vi "PH_ForceSensor.PC Write PSDB.vi"(0 "i ref in":refnum<vi>, 5 "error IO":errorcluster) -> (14 "i ref out":refnum<vi>, 19 "error out":errorcluster)   [LabVIEW 2014, in "PH_ForceSensor.lvlib"]
doc: "This is the proc case which writes data to the PHELIX shot data base."
uses:
  PH_ForceSensor.lvlib
  PH_Basics/PH_PSDBWriter/PH_PSDBWriter.lvlib
  PH_Basics/PH_StatusHandler/PH_StatusHandler.lvlib
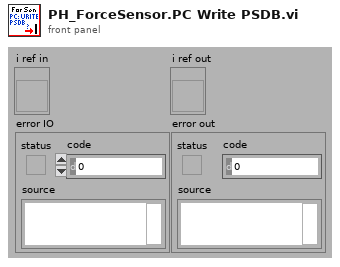
[diagram p1: front panel]
types:
  T1 = typedef "PH_PSDBWriter.lvlib/PH_PSDBWriter.String dataset.ctl" = cluster{"name":string, "data":string, "unit":string}
  T2 = typedef "PH_ForceSensor.lvlib/PH_ForceSensor.i attribute.ctl" = cluster{"GUI Refs":T3, "Rawvalues":T4, "Offsets [µV]":T4, "Scalings [mV/V]":T4, "Forces [N]":T4, "Supply Voltage [V]":dbl, "Full Force [N]":dbl, "Ranges [N]":cluster{"Low Energy":cluster{"Upper Limit":dbl, "Lower Limit":dbl}, "High Energy":cluster{"Upper Limit":dbl, "Lower Limit":dbl}}}
  T3 = typedef "PH_ForceSensor.lvlib/PH_ForceSensor.GUI Refs.ctl" = cluster{"Delete":refnum<vi>, "Rawvalues":refnum<vi>, "Offsets [µV]":refnum<vi>, "Sensor Values [µV]":refnum<vi>, "Scalings [mV/V]":refnum<vi>, "Supply Voltage [V]":refnum<vi>, "Full Force [N]":refnum<vi>, "Forces [N]":refnum<vi>, "Graph Differential Forces":refnum<vi>, "Graph Absolute Forces":refnum<vi>, "Ranges [N]":refnum<vi>}
  T4 = typedef "PH_ForceSensor.lvlib/PH_ForceSensor.Dataset.ctl" = cluster{"top front":dbl, "top back":dbl, "bottom front":dbl, "bottom back":dbl}
  T5 = typedef "PH_PSDBWriter.lvlib/PH_PSDBWriter.Numeric dataset.ctl" = cluster{"name":string, "data":dbl, "unit":string}
  T6 = typedef "PH_PSDBWriter.lvlib/PH_PSDBWriter.PSDB Dataset.ctl" = cluster{"Version":i32, "2D data Input":T7[], "Boolean Input":T9[], "Image Input":T10[], "Numeric Input":T5[], "String Input":T1[]}
  T7 = typedef "PH_PSDBWriter.lvlib/PH_PSDBWriter.2D dataset.ctl" = cluster{"name":string, "data":dbl[][], "axis description":T8}
  T8 = typedef "PSDB.lvlib/PSDB_AxisDescription.ctl" = cluster{"x axis label":string, "y axis label":string, "x axis unit":string, "y axis unit":string}
  T9 = typedef "PH_PSDBWriter.lvlib/PH_PSDBWriter.Boolean dataset.ctl" = cluster{"name":string, "data":bool, "unit":string}
  T10 = typedef "PH_PSDBWriter.lvlib/PH_PSDBWriter.Image dataset.ctl" = cluster{"name":string, "data":T11, "unit":string}
  T11 = typedef "IMAQ Image.ctl" = refnum<image>
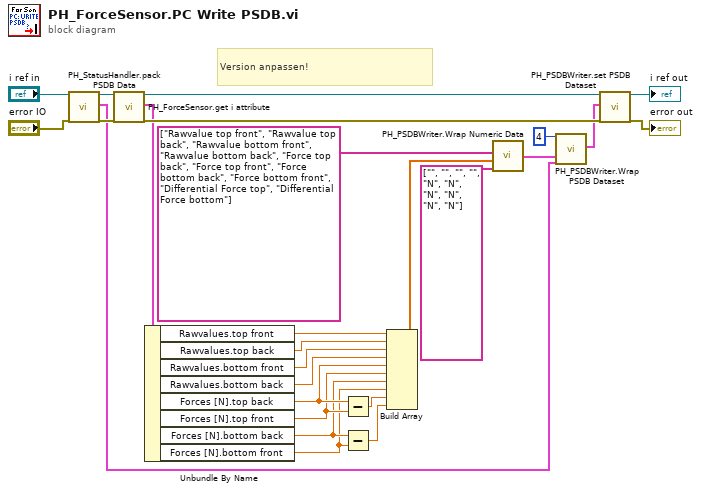
[diagram p0: block diagram]
diagram:
  # "Version anpassen!"
  n1 = call "PH_StatusHandler.pack PSDB Data.vi"("VI in"="i ref in", "error in (no error)"="error IO") -> ("VI out"=w2:refnum<vi>, "PSDB String Data Array"=w1:T1[], "error out"=w4:errorcluster)  [unwired: 15 in]
  n2 = call "PH_ForceSensor.get i attribute.vi"("i ref in"=w2, "error in (no error)"=w4) -> ("i ref out"=w24:refnum<vi>, "i attribute"=w18:T2, "error out"=w26:errorcluster)  [unwired: 15 in]
  n3 = Unbundle By Name(w18) -> ("Rawvalues.top front"=w17:dbl, "Rawvalues.top back"=w16:dbl, "Rawvalues.bottom front"=w15:dbl, "Rawvalues.bottom back"=w14:dbl, "Forces [N].top back"=w13:dbl, "Forces [N].top front"=w12:dbl, "Forces [N].bottom back"=w11:dbl, "Forces [N].bottom front"=w10:dbl)
  n4 = Subtract(x=w13, y=w12) -> (x-y=w9:dbl)
  n5 = Subtract(x=w11, y=w10) -> (x-y=w8:dbl)
  n6 = Build Array(w17, w16, w15, w14, w13, w12, w11, w10, w9, w8) -> (w7:dbl[])
  n7 = call "PH_PSDBWriter.Wrap Numeric Data.vi"("Unit Array"=string[] ["", "", "", "", "N", "N", "N", "N", "N", "N"] ("Name Array"), "Data Array"=w7, "Name Array"=string[] ["Rawvalue top front", "Rawvalue top back", "Rawvalue bottom front", "Rawvalue bottom back", "Force top back", "Force top front", "Force bottom back", "Force bottom front", "Differential Force top", "Differential Force bottom"]) -> ("PSDB Numeric Data Array"=w19:T5[])  [unwired: 1 in]
  n8 = call "PH_PSDBWriter.Wrap PSDB Dataset.vi"("Version"=4, "Numeric Input"=w19, "String Input"=w1) -> ("PSDB Dataset"=w22:T6)  [unwired: 16 in]
  n9 = call "PH_PSDBWriter.set PSDB Dataset.vi"("VI in"=w24, "PSDB Dataset"=w22, "error in (no error)"=w26) -> ("VI out"=→"i ref out":refnum<vi>, "error out"=→"error out":errorcluster)  [unwired: 15 in]
